vi "UTILITY Custom VISA Name.vi"(7 "Default VISA Name":refnum<visa-resource-name>="COM3", 8 "Error In":errorcluster, 11 "Input Name (String)":string) -> (0 "Error Out":errorcluster, 3 "Name (VISA)":refnum<visa-resource-name>)   [LabVIEW 2018]
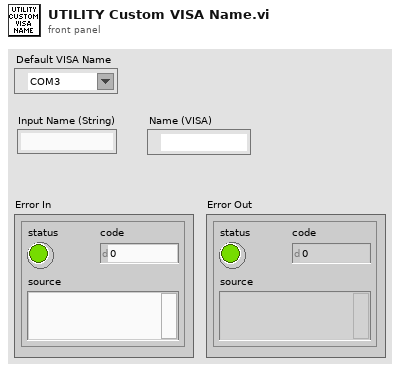
[diagram p1: front panel]
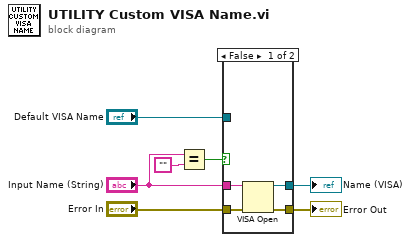
[diagram p0: block diagram]
diagram:
  n1 = Equal?(x="Input Name (String)", y="") -> (x = y?=w5:bool)
  n2 = case shown="False" w5 {
    tunnel: [w10 w12] -> w6
    tunnel: "Input Name (String)" -> [w11 _]
    tunnel: "Error In" -> [w9 w13]
    tunnel: [w8 w13] -> w2
    tunnel: "Default VISA Name" -> [_ w12]
    frame False {
      n3 = VISA Open(error in (no error)=w9, VISA resource name=w11) -> (VISA resource name=w10:refnum<visa-resource-name>, error out=w8:errorcluster)  [unwired: 3 in]
    }
    frame True {
    }
  }
  "Name (VISA)" <- w6
  "Error Out" <- w2
